vi "Part 2.vi"(11 "Input":string) -> (3 "Output":i64)   [LabVIEW 2021]
uses:
  <userlib>/_OpenG.lib/string/string.llb/Convert EOLs (String)__ogtk.vi
  <userlib>/_OpenG.lib/array/array.llb/Delete Elements from 1D Array (I32)__ogtk.vi
panel:
  out "Array":i32[](array[numeric])
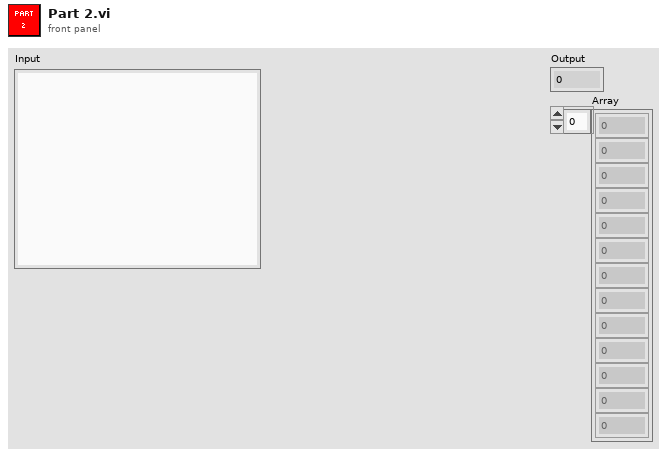
[diagram p1: front panel]
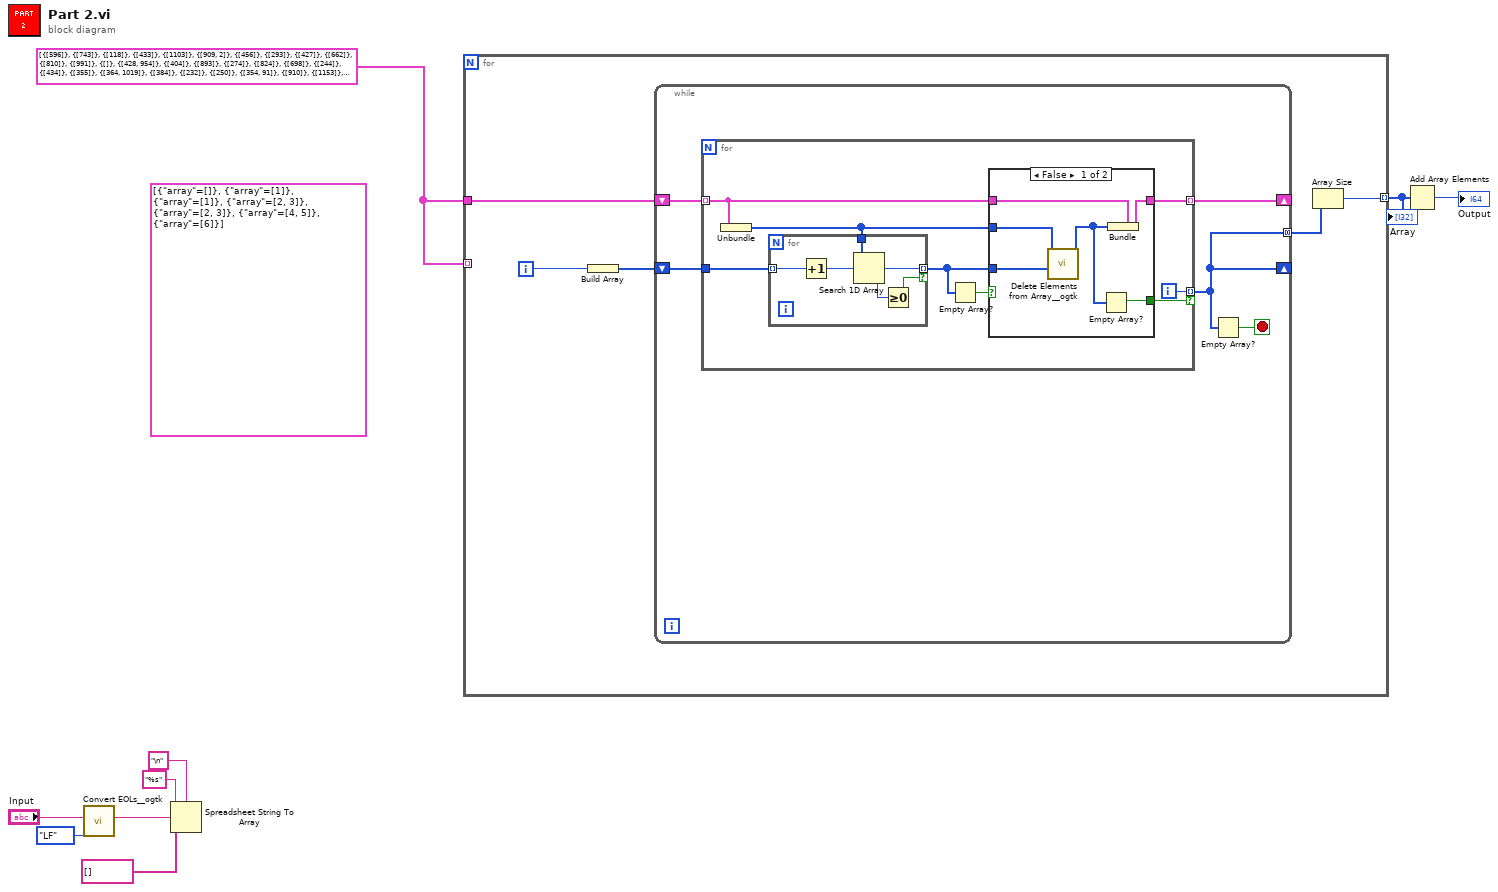
[diagram p0: block diagram]
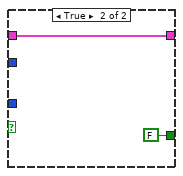
[diagram p2: hidden frame]
diagram:
  (unwired) cluster{"array":i32[]}[] [{"array"=[]}, {"array"=[1]}, {"array"=[1]}, {"array"=[2, 3]}, {"array"=[2, 3]}, {"array"=[4, 5]}, {"array"=[6]}] ("Array")
  w1 = cluster{"array":i32[]}[] [{"array"=[596]}, {"array"=[743]}, {"array"=[118]}, {"array"=[433]}, {"array"=[1103]}, {"array"=[909, 2]}, {"array"=[456]}, {"array"=[293]}, {"array"=[427]}, {"array"=[662]}, {"array"=[810]}, {"array"=[991]}, {"array"=[]}, {"array"=[428, 954]}, {"array"=[404]}, {"array"=[893]}, {"array"=[274]}, {"array"=[824]}, {"array"=[698]}, {"array"=[244]}, {"array"=[434]}, {"array"=[355]}, {"array"=[364, 1019]}, {"array"=[384]}, {"array"=[232]}, {"array"=[250]}, {"array"=[354, 91]}, {"array"=[910]}, {"array"=[1153]}, {"array"=[1001, 872]}, {"array"=[132]}, {"array"=[282]}, {"array"=[47]}, {"array"=[402]}, {"array"=[]}, {"array"=[955]}, {"array"=[265]}, {"array"=[918]}, {"array"=[15]}, {"array"=[989]}, {"array"=[987]}, {"array"=[321]}, {"array"=[266]}, {"array"=[816]}, {"array"=[1025]}, {"array"=[735]}, {"array"=[353]}, {"array"=[7]}, {"array"=[1095]}, {"array"=[51]}, {"array"=[689]}, {"array"=[920]}, {"array"=[589]}, {"array"=[888]}, {"array"=[548]}, {"array"=[514]}, {"array"=[903]}, {"array"=[756]}, {"array"=[618]}, {"array"=[952]}, {"array"=[580]}, {"array"=[682]}, {"array"=[71]}, {"array"=[]}, {"array"=[1070]}, {"array"=[713]}, {"array"=[299]}, {"array"=[970]}, {"array"=[116]}, {"array"=[502]}, {"array"=[715]}, {"array"=[1207]}, {"array"=[1076]}, {"array"=[1050]}, {"array"=[392]}, {"array"=[220]}, {"array"=[73]}, {"array"=[312]}, {"array"=[1038]}, {"array"=[562]}, {"array"=[158]}, {"array"=[231]}, {"array"=[398]}, {"array"=[605]}, {"array"=[720]}, {"array"=[1087]}, {"array"=[25]}, {"array"=[256]}, {"array"=[294, 1017]}, {"array"=[696]}, {"array"=[635]}, {"array"=[526]}, {"array"=[354]}, {"array"=[707]}, {"array"=[863]}, {"array"=[1025]}, {"array"=[634, 476, 831]}, {"array"=[822]}, {"array"=[858]}, {"array"=[826]}, {"array"=[505]}, {"array"=[27]}, {"array"=[1049, 590]}, {"array"=[1171]}, {"array"=[37]}, {"array"=[1101]}, {"array"=[202]}, {"array"=[1052]}, {"array"=[350]}, {"array"=[7]}, {"array"=[895]}, {"array"=[578]}, {"array"=[762]}, {"array"=[883]}, {"array"=[862]}, {"array"=[1198]}, {"array"=[296]}, {"array"=[678]}, {"array"=[983]}, {"array"=[371, 524]}, {"array"=[128]}, {"array"=[1003, 802]}, {"array"=[1054]}, {"array"=[1079]}, {"array"=[292]}, {"array"=[747]}, {"array"=[149]}, {"array"=[1138]}, {"array"=[6]}, {"array"=[59]}, {"array"=[525, 67]}, {"array"=[375]}, {"array"=[1065]}, {"array"=[644]}, {"array"=[848]}, {"array"=[803]}, {"array"=[1209]}, {"array"=[31]}, {"array"=[988]}, {"array"=[1200]}, {"array"=[227]}, {"array"=[1011]}, {"array"=[26]}, {"array"=[1098]}, {"array"=[402]}, {"array"=[1208, 633]}, {"array"=[221, 1178]}, {"array"=[773]}, {"array"=[587]}, {"array"=[793]}, {"array"=[153, 1214]}, {"array"=[915]}, {"array"=[757, 112]}, {"array"=[361]}, {"array"=[980]}, {"array"=[828]}, {"array"=[1053]}, {"array"=[1062]}, {"array"=[992]}, {"array"=[709]}, {"array"=[1114]}, {"array"=[252]}, {"array"=[343]}, {"array"=[332]}, {"array"=[558, 623]}, {"array"=[326]}, {"array"=[11]}, {"array"=[1010]}, {"array"=[1155]}, {"array"=[664]}, {"array"=[162]}, {"array"=[344]}, {"array"=[221, 1178]}, {"array"=[1190]}, {"array"=[212]}, {"array"=[1126]}, {"array"=[19]}, {"array"=[629]}, {"array"=[165, 1193, 751]}, {"array"=[1117]}, {"array"=[95]}, {"array"=[1102]}, {"array"=[367]}, {"array"=[128]}, {"array"=[848]}, {"array"=[591, 9]}, {"array"=[803]}, {"array"=[953]}, {"array"=[560]}, {"array"=[981]}, {"array"=[676]}, {"array"=[1175]}, {"array"=[1057]}, {"array"=[81, 275]}, {"array"=[316]}, {"array"=[581]}, {"array"=[349]}, {"array"=[413]}, {"array"=[1199]}, {"array"=[210]}, {"array"=[1210]}, {"array"=[87]}, {"array"=[]}, {"array"=[829]}, {"array"=[356]}, {"array"=[498]}, {"array"=[1144]}, {"array"=[606]}, {"array"=[1106]}, {"array"=[1211]}, {"array"=[912]}, {"array"=[1067]}, {"array"=[768]}, {"array"=[1126, 1085]}, {"array"=[544]}, {"array"=[311]}, {"array"=[364]}, {"array"=[440]}, {"array"=[659]}, {"array"=[515]}, {"array"=[459]}, {"array"=[1194]}, {"array"=[291]}, {"array"=[956]}, {"array"=[387]}, {"array"=[4, 821]}, {"array"=[353]}, {"array"=[168]}, {"array"=[295]}, {"array"=[1082]}, {"array"=[624]}, {"array"=[1206]}, {"array"=[684]}, {"array"=[442]}, {"array"=[1075]}, {"array"=[267]}, {"array"=[617]}, {"array"=[887]}, {"array"=[1067]}, {"array"=[438]}, {"array"=[154]}, {"array"=[671]}, {"array"=[230]}, {"array"=[948]}, {"array"=[1055, 1033]}, {"array"=[668]}, {"array"=[768, 797]}, {"array"=[196]}, {"array"=[672]}, {"array"=[136]}, {"array"=[662]}, {"array"=[984]}, {"array"=[912]}, {"array"=[477]}, {"array"=[203]}, {"array"=[53]}, {"array"=[355]}, {"array"=[763, 165]}, {"array"=[1156]}, {"array"=[955]}, {"array"=[838]}, {"array"=[731]}, {"array"=[236]}, {"array"=[800]}, {"array"=[1103]}, {"array"=[188]}, {"array"=[1141]}, {"array"=[843]}, {"array"=[1174]}, {"array"=[804]}, {"array"=[794]}, {"array"=[842]}, {"array"=[696]}, {"array"=[1036]}, {"array"=[158]}, {"array"=[1119]}, {"array"=[1081]}, {"array"=[942]}, {"array"=[673]}, {"array"=[1009]}, {"array"=[1009]}, {"array"=[101]}, {"array"=[583]}, {"array"=[717]}, {"array"=[90, 725, 17]}, {"array"=[228]}, {"array"=[604]}, {"array"=[1152]}, {"array"=[640]}, {"array"=[1051]}, {"array"=[478]}, {"array"=[1056]}, {"array"=[190]}, {"array"=[145]}, {"array"=[831]}, {"array"=[1146]}, {"array"=[577]}, {"array"=[737]}, {"array"=[502]}, {"array"=[732]}, {"array"=[674]}, {"array"=[1133, 970]}, {"array"=[505]}, {"array"=[1185]}, {"array"=[]}, {"array"=[94, 514]}, {"array"=[710]}, {"array"=[828]}, {"array"=[786, 711]}, {"array"=[962]}, {"array"=[1055]}, {"array"=[282, 597]}, {"array"=[323]}, {"array"=[1218]}, {"array"=[1058]}, {"array"=[1150]}, {"array"=[239]}, {"array"=[181]}, {"array"=[892]}, {"array"=[84]}, {"array"=[494]}, {"array"=[173]}, {"array"=[1052]}, {"array"=[950]}, {"array"=[866]}, {"array"=[85]}, {"array"=[474]}, {"array"=[534]}, {"array"=[611]}, {"array"=[1186]}, {"array"=[552]}, {"array"=[152]}, {"array"=[1041]}, {"array"=[280]}, {"array"=[417]}, {"array"=[329]}, {"array"=[791]}, {"array"=[26, 586]}, {"array"=[106, 735]}, {"array"=[729]}, {"array"=[598]}, {"array"=[966]}, {"array"=[]}, {"array"=[488, 823]}, {"array"=[41]}, {"array"=[607]}, {"array"=[770]}, {"array"=[148]}, {"array"=[669]}, {"array"=[324]}, {"array"=[508]}, {"array"=[1115]}, {"array"=[520]}, {"array"=[635]}, {"array"=[1073]}, {"array"=[840]}, {"array"=[738]}, {"array"=[746]}, {"array"=[1192]}, {"array"=[137]}, {"array"=[844]}, {"array"=[260]}, {"array"=[970]}, {"array"=[401]}, {"array"=[155]}, {"array"=[50, 148]}, {"array"=[526]}, {"array"=[993]}, {"array"=[1007, 986]}, {"array"=[1149]}, {"array"=[670]}, {"array"=[805]}, {"array"=[592]}, {"array"=[661]}, {"array"=[543, 567]}, {"array"=[396]}, {"array"=[230]}, {"array"=[494]}, {"array"=[833]}, {"array"=[920]}, {"array"=[204]}, {"array"=[893]}, {"array"=[917]}, {"array"=[146]}, {"array"=[340]}, {"array"=[117]}, {"array"=[467]}, {"array"=[497]}, {"array"=[485]}, {"array"=[243]}, {"array"=[962]}, {"array"=[659]}, {"array"=[1120]}, {"array"=[893]}, {"array"=[668]}, {"array"=[105, 752]}, {"array"=[612, 300]}, {"array"=[120]}, {"array"=[241]}, {"array"=[1054]}, {"array"=[378, 666]}, {"array"=[829, 336]}, {"array"=[999, 165]}, {"array"=[634, 476, 831]}, {"array"=[464]}, {"array"=[445]}, {"array"=[374]}, {"array"=[1142]}, {"array"=[852]}, {"array"=[1088]}, {"array"=[551]}, {"array"=[911]}, {"array"=[33]}, {"array"=[1128, 801]}, {"array"=[500]}, {"array"=[742]}, {"array"=[506]}, {"array"=[22, 24]}, {"array"=[164]}, {"array"=[95]}, {"array"=[68]}, {"array"=[727]}, {"array"=[1121]}, {"array"=[1187]}, {"array"=[64]}, {"array"=[977]}, {"array"=[438]}, {"array"=[1028]}, {"array"=[1168]}, {"array"=[489]}, {"array"=[899]}, {"array"=[576]}, {"array"=[66]}, {"array"=[1190]}, {"array"=[867]}, {"array"=[439]}, {"array"=[655, 805]}, {"array"=[1012]}, {"array"=[682, 218]}, {"array"=[902]}, {"array"=[585]}, {"array"=[214]}, {"array"=[697, 648]}, {"array"=[451]}, {"array"=[391]}, {"array"=[111]}, {"array"=[376]}, {"array"=[276]}, {"array"=[1167, 114]}, {"array"=[589]}, {"array"=[990]}, {"array"=[773]}, {"array"=[968]}, {"array"=[345]}, {"array"=[832]}, {"array"=[1066]}, {"array"=[1214]}, {"array"=[564]}, {"array"=[871]}, {"array"=[516]}, {"array"=[285]}, {"array"=[789]}, {"array"=[108, 886]}, {"array"=[109]}, {"array"=[938]}, {"array"=[481]}, {"array"=[929]}, {"array"=[233]}, {"array"=[437]}, {"array"=[]}, {"array"=[35]}, {"array"=[899]}, {"array"=[699]}, {"array"=[151]}, {"array"=[825]}, {"array"=[80, 1047, 730]}, {"array"=[958]}, {"array"=[989]}, {"array"=[]}, {"array"=[451]}, {"array"=[226, 493]}, {"array"=[1046]}, {"array"=[154]}, {"array"=[941]}, {"array"=[642, 123]}, {"array"=[1155]}, {"array"=[537]}, {"array"=[963, 1178]}, {"array"=[1022]}, {"array"=[1023, 607]}, {"array"=[]}, {"array"=[105]}, {"array"=[821]}, {"array"=[262]}, {"array"=[1061]}, {"array"=[932]}, {"array"=[1068]}, {"array"=[578]}, {"array"=[393]}, {"array"=[495]}, {"array"=[293]}, {"array"=[365]}, {"array"=[716]}, {"array"=[853]}, {"array"=[317, 755]}, {"array"=[284]}, {"array"=[288]}, {"array"=[870]}, {"array"=[949]}, {"array"=[641]}, {"array"=[881]}, {"array"=[114]}, {"array"=[248]}, {"array"=[707]}, {"array"=[753]}, {"array"=[420]}, {"array"=[755]}, {"array"=[163, 856]}, {"array"=[778]}, {"array"=[809]}, {"array"=[805]}, {"array"=[1209]}, {"array"=[336]}, {"array"=[413]}, {"array"=[430]}, {"array"=[338]}, {"array"=[455, 700]}, {"array"=[1100]}, {"array"=[588]}, {"array"=[829]}, {"array"=[489]}, {"array"=[964]}, {"array"=[542]}, {"array"=[574]}, {"array"=[865]}, {"array"=[490]}, {"array"=[997]}, {"array"=[10]}, {"array"=[753]}, {"array"=[16]}, {"array"=[735]}, {"array"=[453]}, {"array"=[23]}, {"array"=[600]}, {"array"=[656, 748]}, {"array"=[40]}, {"array"=[878]}, {"array"=[704]}, {"array"=[957]}, {"array"=[846]}, {"array"=[382]}, {"array"=[99]}, {"array"=[1153]}, {"array"=[85]}, {"array"=[173]}, {"array"=[404]}, {"array"=[1086]}, {"array"=[527]}, {"array"=[827]}, {"array"=[475]}, {"array"=[59]}, {"array"=[251, 725]}, {"array"=[759]}, {"array"=[989]}, {"array"=[897]}, {"array"=[1096]}, {"array"=[1176]}, {"array"=[999]}, {"array"=[206]}, {"array"=[501]}, {"array"=[766]}, {"array"=[819]}, {"array"=[98]}, {"array"=[792]}, {"array"=[778]}, {"array"=[851]}, {"array"=[1119]}, {"array"=[1111]}, {"array"=[788]}, {"array"=[222]}, {"array"=[174]}, {"array"=[57]}, {"array"=[140]}, {"array"=[1122]}, {"array"=[]}, {"array"=[250]}, {"array"=[560]}, {"array"=[271]}, {"array"=[1048]}, {"array"=[534]}, {"array"=[1074]}, {"array"=[1018]}, {"array"=[276]}, {"array"=[301]}, {"array"=[658]}, {"array"=[408]}, {"array"=[101]}, {"array"=[502]}, {"array"=[605]}, {"array"=[81]}, {"array"=[296]}, {"array"=[519]}, {"array"=[66]}, {"array"=[211]}, {"array"=[328]}, {"array"=[1135, 288]}, {"array"=[799, 671]}, {"array"=[1187]}, {"array"=[37]}, {"array"=[79]}, {"array"=[564]}, {"array"=[254]}, {"array"=[1169, 1043]}, {"array"=[1076]}, {"array"=[341]}, {"array"=[1068]}, {"array"=[385]}, {"array"=[395]}, {"array"=[111]}, {"array"=[904]}, {"array"=[380, 676, 52]}, {"array"=[307]}, {"array"=[882]}, {"array"=[392, 12]}, {"array"=[85]}, {"array"=[693]}, {"array"=[912]}, {"array"=[7]}, {"array"=[756]}, {"array"=[429]}, {"array"=[800]}, {"array"=[1217]}, {"array"=[955]}, {"array"=[730]}, {"array"=[387]}, {"array"=[11]}, {"array"=[185]}, {"array"=[889]}, {"array"=[166]}, {"array"=[382]}, {"array"=[599]}, {"array"=[207]}, {"array"=[890]}, {"array"=[561]}, {"array"=[890]}, {"array"=[756]}, {"array"=[561]}, {"array"=[617]}, {"array"=[1069]}, {"array"=[854]}, {"array"=[335]}, {"array"=[1077]}, {"array"=[161]}, {"array"=[240]}, {"array"=[575]}, {"array"=[1127]}, {"array"=[881]}, {"array"=[972]}, {"array"=[157]}, {"array"=[505]}, {"array"=[1212]}, {"array"=[705, 62]}, {"array"=[235]}, {"array"=[541]}, {"array"=[23]}, {"array"=[494]}, {"array"=[851]}, {"array"=[309]}, {"array"=[193]}, {"array"=[14]}, {"array"=[934]}, {"array"=[897]}, {"array"=[808]}, {"array"=[241]}, {"array"=[1211]}, {"array"=[920, 342]}, {"array"=[198]}, {"array"=[1111]}, {"array"=[986, 985]}, {"array"=[1072]}, {"array"=[496]}, {"array"=[440]}, {"array"=[380]}, {"array"=[122]}, {"array"=[874]}, {"array"=[390]}, {"array"=[14]}, {"array"=[467]}, {"array"=[971]}, {"array"=[687]}, {"array"=[86]}, {"array"=[646]}, {"array"=[859]}, {"array"=[927]}, {"array"=[550]}, {"array"=[705, 62]}, {"array"=[360]}, {"array"=[866]}, {"array"=[680]}, {"array"=[832]}, {"array"=[327]}, {"array"=[93]}, {"array"=[335, 1131]}, {"array"=[1165]}, {"array"=[682]}, {"array"=[444]}, {"array"=[1100]}, {"array"=[814]}, {"array"=[1118]}, {"array"=[762, 366, 348]}, {"array"=[993]}, {"array"=[1]}, {"array"=[844]}, {"array"=[168]}, {"array"=[416]}, {"array"=[141]}, {"array"=[445]}, {"array"=[1014]}, {"array"=[1001]}, {"array"=[761]}, {"array"=[1122]}, {"array"=[1013]}, {"array"=[691]}, {"array"=[908]}, {"array"=[696]}, {"array"=[1183]}, {"array"=[268]}, {"array"=[790, 813]}, {"array"=[20]}, {"array"=[562]}, {"array"=[917]}, {"array"=[1129]}, {"array"=[131]}, {"array"=[711]}, {"array"=[67]}, {"array"=[998, 463]}, {"array"=[54]}, {"array"=[491]}, {"array"=[320]}, {"array"=[367]}, {"array"=[47]}, {"array"=[797]}, {"array"=[49]}, {"array"=[]}, {"array"=[263]}, {"array"=[175]}, {"array"=[13]}, {"array"=[1127, 443]}, {"array"=[819]}, {"array"=[239]}, {"array"=[623]}, {"array"=[37]}, {"array"=[928]}, {"array"=[35]}, {"array"=[536]}, {"array"=[665]}, {"array"=[1068]}, {"array"=[1116]}, {"array"=[148]}, {"array"=[1001]}, {"array"=[575]}, {"array"=[718]}, {"array"=[558]}, {"array"=[211]}, {"array"=[483]}, {"array"=[1166]}, {"array"=[1200]}, {"array"=[298]}, {"array"=[137]}, {"array"=[258]}, {"array"=[647]}, {"array"=[225]}, {"array"=[480]}, {"array"=[594]}, {"array"=[879]}, {"array"=[519, 575]}, {"array"=[621, 191]}, {"array"=[775]}, {"array"=[834]}, {"array"=[719]}, {"array"=[818]}, {"array"=[931, 650]}, {"array"=[377]}, {"array"=[570]}, {"array"=[26, 586]}, {"array"=[993]}, {"array"=[409]}, {"array"=[1082]}, {"array"=[806]}, {"array"=[757]}, {"array"=[196]}, {"array"=[482]}, {"array"=[63, 925]}, {"array"=[1104]}, {"array"=[465]}, {"array"=[127]}, {"array"=[298]}, {"array"=[827]}, {"array"=[934]}, {"array"=[1209]}, {"array"=[1094]}, {"array"=[781]}, {"array"=[1124]}, {"array"=[533, 716]}, {"array"=[749]}, {"array"=[1024]}, {"array"=[221]}, {"array"=[817, 680]}, {"array"=[1034]}, {"array"=[282]}, {"array"=[379]}, {"array"=[630]}, {"array"=[982]}, {"array"=[186]}, {"array"=[295]}, {"array"=[1113]}, {"array"=[1159]}, {"array"=[637]}, {"array"=[994]}, {"array"=[351]}, {"array"=[603]}, {"array"=[1157]}, {"array"=[963]}, {"array"=[626]}, {"array"=[894]}, {"array"=[518]}, {"array"=[381]}, {"array"=[665]}, {"array"=[329]}, {"array"=[723]}, {"array"=[80, 1047]}, {"array"=[63]}, {"array"=[169]}, {"array"=[901]}, {"array"=[442]}, {"array"=[455, 700]}, {"array"=[1108]}, {"array"=[377, 23]}, {"array"=[501]}, {"array"=[856]}, {"array"=[876]}, {"array"=[1031]}, {"array"=[931]}, {"array"=[1078]}, {"array"=[1181]}, {"array"=[503, 1006]}, {"array"=[782]}, {"array"=[8]}, {"array"=[1069]}, {"array"=[911]}, {"array"=[677]}, {"array"=[20]}, {"array"=[334]}, {"array"=[449]}, {"array"=[606]}, {"array"=[104]}, {"array"=[1121]}, {"array"=[740]}, {"array"=[496]}, {"array"=[632]}, {"array"=[]}, {"array"=[207]}, {"array"=[1170]}, {"array"=[853]}, {"array"=[1123]}, {"array"=[710]}, {"array"=[967]}, {"array"=[377]}, {"array"=[813]}, {"array"=[919]}, {"array"=[1039, 256]}, {"array"=[925]}, {"array"=[830]}, {"array"=[634]}, {"array"=[1191]}, {"array"=[91]}, {"array"=[416]}, {"array"=[310]}, {"array"=[1060]}, {"array"=[1092]}, {"array"=[923]}, {"array"=[455]}, {"array"=[862, 642]}, {"array"=[91]}, {"array"=[179]}, {"array"=[1136]}, {"array"=[932]}, {"array"=[919]}, {"array"=[466]}, {"array"=[1119]}, {"array"=[502]}, {"array"=[826]}, {"array"=[1167]}, {"array"=[333]}, {"array"=[827]}, {"array"=[285]}, {"array"=[1217]}, {"array"=[160]}, {"array"=[483]}, {"array"=[539]}, {"array"=[697, 648]}, {"array"=[1179]}, {"array"=[947]}, {"array"=[1145]}, {"array"=[346]}, {"array"=[31]}, {"array"=[394]}, {"array"=[1074]}, {"array"=[743, 1098]}, {"array"=[]}, {"array"=[771, 1193]}, {"array"=[350]}, {"array"=[435, 278]}, {"array"=[299]}, {"array"=[869]}, {"array"=[273]}, {"array"=[452]}, {"array"=[232]}, {"array"=[337]}, {"array"=[280]}, {"array"=[487]}, {"array"=[210]}, {"array"=[304]}, {"array"=[517, 330]}, {"array"=[71]}, {"array"=[479]}, {"array"=[220]}, {"array"=[1112]}, {"array"=[347]}, {"array"=[394]}, {"array"=[573]}, {"array"=[1132]}, {"array"=[]}, {"array"=[422]}, {"array"=[686]}, {"array"=[809]}, {"array"=[368]}, {"array"=[513]}, {"array"=[538]}, {"array"=[531]}, {"array"=[1025]}, {"array"=[727]}, {"array"=[991, 102]}, {"array"=[1143, 1176]}, {"array"=[1057]}, {"array"=[535]}, {"array"=[785]}, {"array"=[532]}, {"array"=[264]}, {"array"=[474]}, {"array"=[684]}, {"array"=[772]}, {"array"=[26]}, {"array"=[1028]}, {"array"=[892, 100]}, {"array"=[771]}, {"array"=[1017]}, {"array"=[722]}, {"array"=[1184]}, {"array"=[763]}, {"array"=[223]}, {"array"=[209]}, {"array"=[667]}, {"array"=[398]}, {"array"=[1107]}, {"array"=[1009]}, {"array"=[843]}, {"array"=[439, 1036]}, {"array"=[854]}, {"array"=[472]}, {"array"=[990]}, {"array"=[667]}, {"array"=[1180]}, {"array"=[1189, 147]}, {"array"=[229]}, {"array"=[107]}, {"array"=[1114]}, {"array"=[1010]}, {"array"=[301]}, {"array"=[969]}, {"array"=[714]}, {"array"=[757]}, {"array"=[620]}, {"array"=[653]}, {"array"=[546]}, {"array"=[546]}, {"array"=[718]}, {"array"=[449]}, {"array"=[431]}, {"array"=[183]}, {"array"=[93]}, {"array"=[996]}, {"array"=[124]}, {"array"=[104]}, {"array"=[710]}, {"array"=[349]}, {"array"=[355]}, {"array"=[886]}, {"array"=[623]}, {"array"=[190]}, {"array"=[1065]}, {"array"=[1040]}, {"array"=[781]}, {"array"=[1023]}, {"array"=[559]}, {"array"=[358]}, {"array"=[458]}, {"array"=[278]}, {"array"=[557]}, {"array"=[214]}, {"array"=[795]}, {"array"=[298]}, {"array"=[226]}, {"array"=[689]}, {"array"=[1016]}, {"array"=[514]}, {"array"=[145]}, {"array"=[849]}, {"array"=[42]}, {"array"=[959]}, {"array"=[]}, {"array"=[139]}, {"array"=[799]}, {"array"=[406, 1116]}, {"array"=[1030]}, {"array"=[460]}, {"array"=[457]}, {"array"=[916]}, {"array"=[877]}, {"array"=[622]}, {"array"=[82]}, {"array"=[478]}, {"array"=[1064, 384]}, {"array"=[1004]}, {"array"=[650, 74]}, {"array"=[218]}, {"array"=[550]}, {"array"=[1039]}, {"array"=[450]}, {"array"=[1080]}, {"array"=[345]}, {"array"=[1099]}, {"array"=[592]}, {"array"=[1011]}, {"array"=[961]}, {"array"=[457]}, {"array"=[562, 285]}, {"array"=[716]}, {"array"=[534]}, {"array"=[512]}, {"array"=[476, 831]}, {"array"=[629, 58]}, {"array"=[929]}, {"array"=[1144]}, {"array"=[384]}, {"array"=[46]}, {"array"=[30]}, {"array"=[330]}, {"array"=[898]}, {"array"=[]}, {"array"=[652]}, {"array"=[466]}, {"array"=[906]}, {"array"=[146]}, {"array"=[668]}, {"array"=[272]}, {"array"=[607]}, {"array"=[323]}, {"array"=[133]}, {"array"=[946]}, {"array"=[885]}, {"array"=[1128]}, {"array"=[1124]}, {"array"=[693]}, {"array"=[39]}, {"array"=[16]}, {"array"=[1041]}, {"array"=[784]}, {"array"=[25]}, {"array"=[843]}, {"array"=[787]}, {"array"=[378]}, {"array"=[173]}, {"array"=[92]}, {"array"=[613]}, {"array"=[526]}, {"array"=[655]}, {"array"=[914]}, {"array"=[608]}, {"array"=[468]}, {"array"=[1121, 710]}, {"array"=[953]}, {"array"=[345]}, {"array"=[493]}, {"array"=[1084]}, {"array"=[182]}, {"array"=[156]}, {"array"=[49]}, {"array"=[563]}, {"array"=[141]}, {"array"=[299]}, {"array"=[426]}, {"array"=[312]}, {"array"=[604]}, {"array"=[799, 671]}, {"array"=[118]}, {"array"=[815]}, {"array"=[339]}, {"array"=[761]}, {"array"=[169]}, {"array"=[868]}, {"array"=[1039, 256]}, {"array"=[580]}, {"array"=[]}, {"array"=[389]}, {"array"=[445]}, {"array"=[421]}, {"array"=[169]}, {"array"=[407]}, {"array"=[231]}, {"array"=[917]}, {"array"=[1085]}, {"array"=[1134]}, {"array"=[319]}, {"array"=[168]}, {"array"=[613]}, {"array"=[571]}, {"array"=[1094]}, {"array"=[249]}, {"array"=[874]}, {"array"=[1190]}, {"array"=[745]}, {"array"=[472]}, {"array"=[21]}, {"array"=[304]}, {"array"=[629, 58]}, {"array"=[]}, {"array"=[1189]}, {"array"=[937]}, {"array"=[918]}, {"array"=[794]}, {"array"=[119]}, {"array"=[1019]}, {"array"=[523]}, {"array"=[27]}, {"array"=[286]}, {"array"=[345]}, {"array"=[611]}, {"array"=[1029]}, {"array"=[933]}, {"array"=[537]}, {"array"=[549]}, {"array"=[638]}, {"array"=[942]}, {"array"=[195]}, {"array"=[968]}, {"array"=[204]}, {"array"=[1142]}, {"array"=[565, 860]}, {"array"=[121]}, {"array"=[471]}, {"array"=[210]}, {"array"=[1147]}, {"array"=[1051]}, {"array"=[1089]}, {"array"=[432]}, {"array"=[883]}, {"array"=[434]}, {"array"=[592]}, {"array"=[454]}, {"array"=[]}, {"array"=[266]}, {"array"=[476]}, {"array"=[54]}, {"array"=[52]}, {"array"=[1019]}, {"array"=[24]}, {"array"=[948]}, {"array"=[598, 70]}, {"array"=[130]}, {"array"=[2]}, {"array"=[940]}, {"array"=[1002]}, {"array"=[1109]}, {"array"=[957]}, {"array"=[905]}, {"array"=[928]}, {"array"=[631]}, {"array"=[663, 221]}, {"array"=[506]}, {"array"=[594]}, {"array"=[897]}, {"array"=[558, 623]}, {"array"=[1141]}, {"array"=[1212, 463]}, {"array"=[749]}, {"array"=[51]}, {"array"=[1126]}, {"array"=[143]}, {"array"=[1162]}, {"array"=[1066]}, {"array"=[776]}, {"array"=[847]}, {"array"=[726]}, {"array"=[199]}, {"array"=[263]}, {"array"=[419]}, {"array"=[521]}, {"array"=[344]}, {"array"=[]}, {"array"=[8]}, {"array"=[108, 886]}, {"array"=[1216]}, {"array"=[757]}, {"array"=[913]}, {"array"=[224]}, {"array"=[899, 765]}, {"array"=[318]}] ("Array")
  n1 = call-poly <userlib>:"Convert EOLs__ogtk.vi"("Convert to:"=enum16{"CR", "LF", "CRLF"}."LF", "String in"="Input") -> ("String out"=w5:string)  [unwired: 9 in]
  n2 = Spreadsheet String To Array(delimiter (Tab)="\n", format string="%s", spreadsheet string=w5, array type (2D Dbl)=string[] []) -> ()  [unwired: 1 out]
  n3 = for {
    tunnel: w1 -> [_] mode=indexing
    tunnel: w1 -> [w14]
    tunnel: [w11] -> w3 mode=indexing
    i -> [w10]
    n4 = Build Array(w10) -> (w13:i32[])
    n5 = while {
      shift-right: [w16] -> _
      shift-left: w13 -> [w18]
      tunnel: [w16] -> w12 mode=concatenating
      shift-right: [w15] -> _
      shift-left: w14 -> [w19]
      stop <- w17 stop-if-true
      n6 = for {
        tunnel: w19 -> [w26] mode=indexing
        tunnel: w18 -> [w27]
        tunnel: [w25] -> w16 mode=indexing if=w23
        tunnel: [w22] -> w15 mode=indexing
        i -> [w25]
        n7 = Unbundle(w26) -> ("array"=w24:i32[])
        n8 = for {
          tunnel: w27 -> [w32] mode=indexing
          tunnel: w24 -> [w31]
          tunnel: [w29] -> w20 mode=indexing if=w30
          n9 = Increment(x=w32) -> (x+1=w28:i32)
          n10 = Search 1D Array(1D array=w31, element=w28) -> (index of element=w29:i32)  [unwired: 1 in]
          n11 = Greater Or Equal To 0?(x=w29) -> (x >= 0?=w30:bool)
        }
        n12 = Empty Array?(array=w20) -> (empty?=w21:bool)
        n13 = case shown="False" w21 {
          tunnel: w26 -> [w38 w40]
          tunnel: w24 -> [w37 _]
          tunnel: [w34 FALSE] -> w23
          tunnel: [w36 w40] -> w22
          tunnel: w20 -> [w35 _]
          frame False {
            n14 = call-poly <userlib>:"Delete Elements from Array__ogtk.vi"("indices"=w35, "array"=w37) -> ("array w/ subset deleted"=w33:i32[])  [unwired: 8 in, 1 out]
            n15 = Empty Array?(array=w33) -> (empty?=w34:bool)
            n16 = Bundle(cluster=w38, "array"=w33) -> (w36:cluster{"array":i32[]})
          }
          frame True {
          }
        }
      }
      n17 = Empty Array?(array=w16) -> (empty?=w17:bool)
    }
    n18 = Array Size(array=w12) -> (size(s)=w11:i32)
  }
  "Array" <- w3
  n19 = Add Array Elements(numeric array=w3) -> (sum=→"Output":i32)
